vi "InitConnection.vi"(8 "ErrorIn":errorcluster) -> (0 "ErrorOut":errorcluster, 3 "OutConnection":T1)   [LabVIEW 2019]
uses:
  C:/Users/yasav/Downloads/prev_robocad/robocadSimLVFolder/assemblies/LibraryForLabVIEW.dll
  assemblies/LibraryForLabVIEW.dll
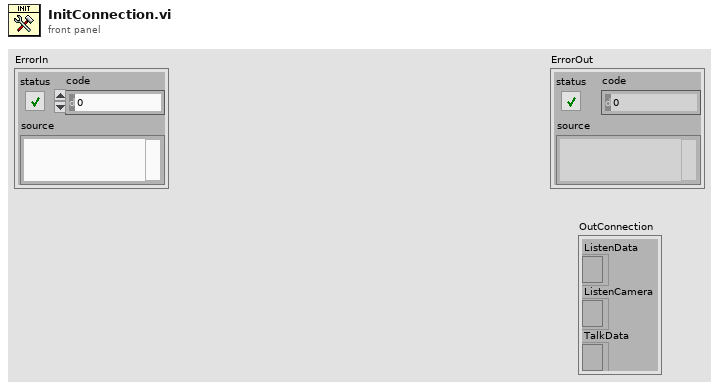
[diagram p1: front panel]
types:
  T1 = cluster{"ListenData":refnum<k24>, "ListenCamera":refnum<k24>, "TalkData":refnum<k24>}
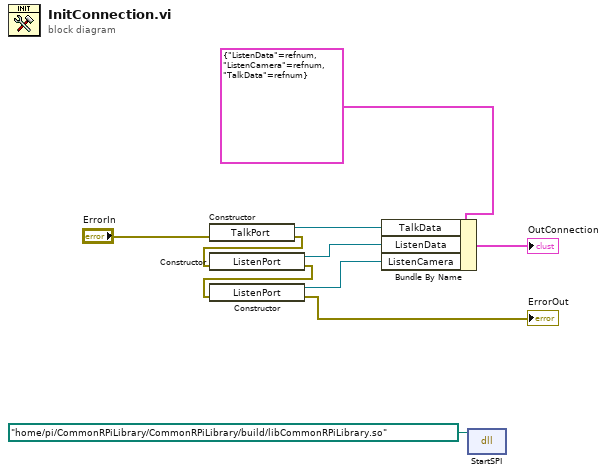
[diagram p0: block diagram]
diagram:
  n1 = constructor class="TalkPort"(error in="ErrorIn") -> (reference out=w8:refnum<k24>, error out=w3:errorcluster)  [unwired: 2 in, 1 out]
  n2 = constructor class="ListenPort"(error in=w3) -> (reference out=w6:refnum<k24>, error out=w4:errorcluster)  [unwired: 2 in, 1 out]
  n3 = constructor class="ListenPort"(error in=w4) -> (reference out=w5:refnum<k24>, error out=→"ErrorOut":errorcluster)  [unwired: 2 in, 1 out]
  n4 = Bundle By Name(cluster=T1 {"ListenData"=refnum, "ListenCamera"=refnum, "TalkData"=refnum}, "TalkData"=w8, "ListenData"=w6, "ListenCamera"=w5) -> (→"OutConnection":T1)
  n5 = dll-call lib="?" fn="StartSPI"(path in=path "/home/pi/CommonRPiLibrary/CommonRPiLibrary/build/libCommonRPiLibrary.so") -> ()  [unwired: 3 in, 2 out]
